vi "Spiral Matrix.vi"(11 "Numeric":i32) -> (3 "Array":i32[][](array[numeric]))   [LabVIEW 2014]
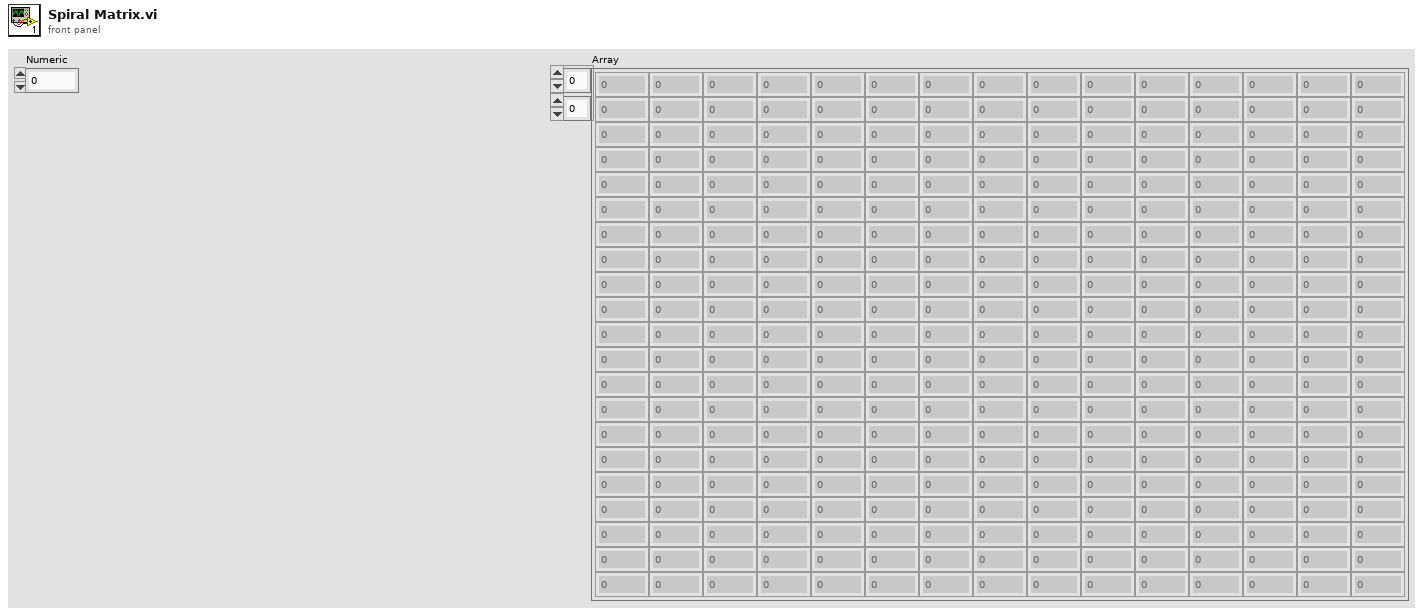
[diagram p1: front panel]
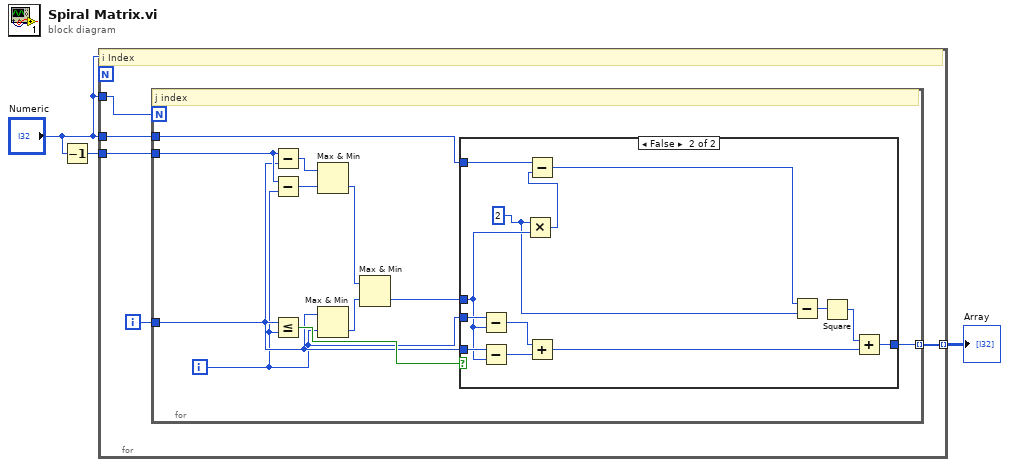
[diagram p0: block diagram]
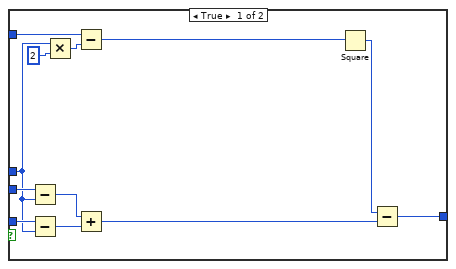
[diagram p2: hidden frame]
diagram:
  n1 = Decrement(x="Numeric") -> (x-1=w3:i32)
  n2 = for {
    N: "Numeric" -> [_]
    tunnel: "Numeric" -> [w8]
    tunnel: w3 -> [w6]
    tunnel: "Numeric" -> [w5]
    tunnel: [w4] -> w1 mode=indexing
    i -> [w7]
    # "i Index"
    n3 = for {
      N: w8 -> [_]
      tunnel: w7 -> [w11]
      tunnel: w6 -> [w19]
      tunnel: w5 -> [w12]
      tunnel: [w9] -> w4 mode=indexing
      i -> [w10]
      # "j index"
      n4 = Subtract(x=w19, y=w11) -> (x-y=w18:i32)
      n5 = Subtract(x=w19, y=w10) -> (x-y=w17:i32)
      n6 = Less Or Equal?(x=w11, y=w10) -> (x <= y?=w14:bool)
      n7 = Max & Min(x=w18, y=w17) -> (min(x,y)=w16:i32)  [unwired: 1 out]
      n8 = Max & Min(x=w11, y=w10) -> (min(x,y)=w15:i32)  [unwired: 1 out]
      n9 = Max & Min(x=w16, y=w15) -> (min(x,y)=w13:i32)  [unwired: 1 out]
      n10 = case shown="False" w14 {
        tunnel: w13 -> [w23 w34]
        tunnel: w12 -> [w31 w44]
        tunnel: w11 -> [w30 w43]
        tunnel: w10 -> [w29 w42]
        tunnel: [w24 w38] -> w9
        frame True {
          n11 = Subtract(x=w29, y=w23) -> (x-y=w27:i32)
          n12 = Subtract(x=w30, y=w23) -> (x-y=w25:i32)
          n13 = Multiply(x=w23, y=2) -> (x*y=w21:i32)
          n14 = Subtract(x=w31, y=w21) -> (x-y=w20:i32)
          n15 = Add(x=w27, y=w25) -> (x+y=w26:i32)
          n16 = Square(x=w20) -> (x^2=w28:i32)
          n17 = Subtract(x=w28, y=w26) -> (x-y=w24:i32)
        }
        frame False {
          w32 = 2 ("y")
          n18 = Subtract(x=w42, y=w34) -> (x-y=w41:i32)
          n19 = Subtract(x=w43, y=w34) -> (x-y=w39:i32)
          n20 = Multiply(x=w32, y=w34) -> (x*y=w33:i32)
          n21 = Subtract(x=w44, y=w33) -> (x-y=w37:i32)
          n22 = Add(x=w41, y=w39) -> (x+y=w40:i32)
          n23 = Subtract(x=w37, y=w32) -> (x-y=w36:i32)
          n24 = Square(x=w36) -> (x^2=w35:i32)
          n25 = Add(x=w35, y=w40) -> (x+y=w38:i32)
        }
      }
    }
  }
  "Array" <- w1
